vi "Sequencer Main - Copy.vi"() -> ()   [LabVIEW 2018] (continued)
                                frame #0 {
                                n2354 = global read "Global Variable.vi" "COM Port FTDI RS232"() -> (w4643:refnum<visa-resource-name>)
                                n2355 = global read "Global Variable.vi" "Wr PID"() -> (w4640:string)
                                n2356 = call "ADB-Serial_WrRd.vi"("Timeout(Sec)"=1.0, "PassString"=w4640, "Command"="getPID", "ComPort"=w4643) -> ("error out"=w4645:errorcluster, "PASS"=w4646:bool, "received"=w4644:string)  [unwired: 5 in]
                                n2357 = invoke on="Serial CMD Mon" class="Str" method="Append String"("string"=w4644) -> ()  [unwired: 3 in, 4 out]
                                n2358 = Wait (ms)(milliseconds to wait=u32 250) -> ()  [unwired: 1 out]
                                }
                                frame #1 {
                                n2359 = in-place {
                                in-place-border: w4653 -> [w4661]
                                in-place-border: [w4661] -> w4652
                                in-place-border: [w4662] -> w4648
                                in-place-border: w4651 -> [w4659]
                                n2360 = Match Pattern(string=w4659, regular expression="PID:" ("search string/char (-)")) -> (after substring=w4658:string)  [unwired: 1 in, 3 out]
                                n2361 = String Subset(string=w4658, offset (0)=1, length (rest)=13 ("length (rest)")) -> (substring=w4662:string)
                                n2362 = global write "Global Variable.vi" "Rd PID"(w4662) -> ()
                                }
                                n2363 = global read "Global Variable.vi" "Array Errors"() -> (w4657:errorcluster[])
                                n2364 = case shown="False" w4650 {
                                tunnel: [enum16{"Idle", "PASS", "FALSE"}."FALSE" ("Step Test Result") enum16{"Idle", "PASS", "FALSE"}."PASS" ("Step Test Result")] -> w4654
                                frame False {
                                # "Step TEST Result"
                                }
                                frame True {
                                # "Step TEST Result"
                                }
                                }
                                n2365 = Replace Array Subset(array=w4657, new element=w4652, index=3) -> (w4656:errorcluster[])
                                n2366 = global write "Global Variable.vi" "Array Errors"(w4656) -> ()
                                n2367 = Concatenate Strings("Read PID: " ("string"), w4648) -> (w4647:string)
                                }
                              }
                            }
                            frame "setpid" {
                              n2368 = flat-sequence {
                                tunnel: [w4680] -> w4671
                                tunnel: [w4722] -> w4673
                                tunnel: [w4721] -> w4672
                                tunnel: w4671 -> [w4716]
                                tunnel: [w4718] -> w4669
                                tunnel: [w4717] -> w4667
                                frame #0 {
                                w4691 = 5
                                # "Replace Space to 0"
                                # "YY: Year 00-99\nWW: Week 01-53\nSS: Supplier ID (SVI: 04)\nxx: Spare\nNNNNN: Ser Number"
                                # "default"
                                n2369 = local read "Barcode"() -> (w4679:string)
                                n2370 = global write "Global Variable.vi" "Wr PID"("") -> ()
                                n2371 = String Length(string=w4679) -> (length=w4690:i32)
                                n2372 = Greater?(x=w4690, y=w4691) -> (0:w4692:bool)
                                n2373 = case shown="True" w4692 {
                                tunnel: w4679 -> [_ w4715]
                                tunnel: w4691 -> [_ w4713]
                                tunnel: w4690 -> [_ w4714]
                                tunnel: "1111040011111" ("ADB_PID") -> [w4695 w4711]
                                tunnel: [w4695 w4701] -> w4685
                                frame False {
                                }
                                frame True {
                                w4697 = "%2d" ("format string")
                                n2374 = Subtract(x=w4714, y=w4713) -> (x-y=w4712:i32)
                                n2375 = call "Calc_ISO_WeekNumber.vi"() -> ("ISO week number"=w4696:i32, "SBZ year 2 digits"=w4700:i32)  [unwired: 5 in, 5 out]
                                n2376 = String Subset(string=w4715, offset (0)=w4712, length (rest)=w4713) -> (substring=w4710:string)
                                n2377 = Format Into String(format string=w4697, w4700) -> (resulting string=w4699:string)  [unwired: 2 in, 1 out]
                                n2378 = Replace Substring(2:5 ("length (len. of substring)"), 3:8 ("offset (0)"), 4:w4710, 5:w4711) -> (1:w4707:string)  [unwired: 1 out]
                                n2379 = Format Into String(format string=w4697, w4696) -> (resulting string=w4698:string)  [unwired: 2 in, 1 out]
                                n2380 = Replace Substring(2:2 ("offset (0)"), 3:0 ("offset (0)"), 4:w4699, 5:w4707) -> (1:w4702:string)  [unwired: 1 out]
                                n2381 = Replace Substring(2:2 ("offset (0)"), 3:2 ("offset (0)"), 4:w4698, 5:w4702) -> (1:w4701:string)  [unwired: 1 out]
                                }
                                }
                                n2382 = local read "Barcode\nDefault"() -> (w4678:bool)
                                n2383 = call <vilib>:"Space Constant.vi"() -> ("String"=w4683:string)
                                n2384 = call <vilib>:"Search and Replace Pattern.vi"("string"=w4685, "regular expression (\"\")"=w4683, "replace string (\"\")"="0" ("replace string (\"\")")) -> ("result string"=w4681:string)  [unwired: 2 in, 1 out]
                                n2385 = case shown="False" w4678 {
                                tunnel: w4681 -> [_ w4694]
                                tunnel: [w4693 w4694] -> w4680
                                tunnel: w4679 -> [w4693 _]
                                frame False {
                                }
                                frame True {
                                }
                                }
                                n2386 = Concatenate Strings("Calculated PID: ", w4680, "\r\n") -> (w4682:string)
                                n2387 = invoke on="Serial CMD Mon" class="Str" method="Append String"("string"=w4682) -> ()  [unwired: 3 in, 4 out]
                                }
                                frame #1 {
                                n2388 = global read "Global Variable.vi" "COM Port FTDI RS232"() -> (w4720:refnum<visa-resource-name>)
                                n2389 = call "ADB-SetPID.vi"("ADB_PID"=w4716, "ComPort"=w4720) -> ("error out"=w4721:errorcluster, "Wr PID"=w4718:string, "PASS"=w4722:bool, "received"=w4717:string)  [unwired: 6 in]
                                n2390 = invoke on="Serial CMD Mon" class="Str" method="Append String"("string"=w4717) -> ()  [unwired: 3 in, 4 out]
                                n2391 = global write "Global Variable.vi" "Wr PID"(w4718) -> ()
                                n2392 = Wait (ms)(milliseconds to wait=u32 5000) -> ()  [unwired: 1 out]
                                }
                              }
                              n2393 = global read "Global Variable.vi" "Array Errors"() -> (w4676:errorcluster[])
                              n2394 = case shown="False" w4673 {
                                tunnel: [enum16{"Idle", "PASS", "FALSE"}."FALSE" ("Step Test Result") enum16{"Idle", "PASS", "FALSE"}."PASS" ("Step Test Result")] -> w4677
                                frame False {
                                # "Step TEST Result"
                                }
                                frame True {
                                # "Step TEST Result"
                                }
                              }
                              n2395 = Replace Array Subset(array=w4676, new element=w4672, index=5) -> (w4675:errorcluster[])
                              n2396 = Concatenate Strings("Write PID: " ("string"), w4669) -> (w4668:string)
                              n2397 = global write "Global Variable.vi" "Array Errors"(w4675) -> ()
                            }
                            frame "recvtest" {
                              # "Param 1-4"
                              # "Cmd"
                              n2398 = flat-sequence {
                                tunnel: [w4758] -> w4742
                                tunnel: [w4757] -> w4741
                                tunnel: [w4756] -> w4740
                                tunnel: w4739 -> [w4755]
                                tunnel: w4738 -> [w4754]
                                tunnel: w4737 -> [w4753]
                                tunnel: w4736 -> [w4752]
                                tunnel: [w4751] -> w4735
                                tunnel: [w4750] -> w4734
                                tunnel: [w4749] -> w4733
                                tunnel: [w4748] -> w4732
                                tunnel: [w4747] -> w4731
                                tunnel: [w4746] -> w4730
                                tunnel: [w4745] -> w4729
                                tunnel: [w4744] -> w4728
                                tunnel: w4742 -> [w4797]
                                tunnel: w4741 -> [w4816]
                                tunnel: [w4817] -> w4727
                                tunnel: w4740 -> [w4795]
                                tunnel: w4735 -> [w4807]
                                tunnel: w4734 -> [w4806]
                                tunnel: w4733 -> [w4805]
                                tunnel: w4732 -> [w4804]
                                tunnel: w4731 -> [w4803]
                                tunnel: w4730 -> [w4802]
                                tunnel: w4729 -> [w4801]
                                tunnel: w4728 -> [w4800]
                                tunnel: [w4796] -> w4726
                                tunnel: [w4795] -> w4725
                                frame #0 {
                                w4743 = "%f" ("format string")
                                n2399 = for {
                                N: 1 -> [_]
                                tunnel: [w4791] -> w4758
                                tunnel: [w4790] -> w4757
                                tunnel: [w4789] -> w4756
                                stop <- w4791 stop-if-true
                                n2400 = global read "Global Variable.vi" "COM Port FTDI RS232"() -> (w4794:refnum<visa-resource-name>)
                                n2401 = call "ADB-Serial_WrRd.vi"("Timeout(Sec)"=5.0, "PassString"="Chuck(3):", "Command"="recvtest", "ComPort"=w4794) -> ("error out"=w4790:errorcluster, "PASS"=w4791:bool, "received"=w4789:string)  [unwired: 5 in]
                                n2402 = invoke on="Serial CMD Mon" class="Str" method="Append String"("string"=w4789) -> ()  [unwired: 3 in, 4 out]
                                }
                                n2403 = in-place {
                                in-place-border: w4755 -> [w4787]
                                in-place-border: [w4783] -> w4751
                                in-place-border: [w4782] -> w4750
                                in-place-border: w4743 -> [w4781]
                                # "max"
                                # "min"
                                # "LMS RX -> k_est"
                                n2404 = Match Pattern(string=w4787, regular expression=":") -> (before substring=w4785:string, after substring=w4784:string)  [unwired: 1 in, 2 out]
                                n2405 = Scan From String(format string=w4781, input string=w4785) -> (output 1=w4783:dbl)  [unwired: 3 in, 3 out]
                                n2406 = Scan From String(format string=w4781, input string=w4784) -> (output 1=w4782:dbl)  [unwired: 3 in, 3 out]
                                }
                                n2407 = in-place {
                                in-place-border: w4754 -> [w4780]
                                in-place-border: [w4776] -> w4749
                                in-place-border: [w4775] -> w4748
                                in-place-border: w4743 -> [w4774]
                                # "max"
                                # "min"
                                # "LMS RX -> I_est"
                                n2408 = Match Pattern(string=w4780, regular expression=":") -> (before substring=w4778:string, after substring=w4777:string)  [unwired: 1 in, 2 out]
                                n2409 = Scan From String(format string=w4774, input string=w4778) -> (output 1=w4776:dbl)  [unwired: 3 in, 3 out]
                                n2410 = Scan From String(format string=w4774, input string=w4777) -> (output 1=w4775:dbl)  [unwired: 3 in, 3 out]
                                }
                                n2411 = in-place {
                                in-place-border: w4753 -> [w4773]
                                in-place-border: [w4769] -> w4747
                                in-place-border: [w4768] -> w4746
                                in-place-border: w4743 -> [w4767]
                                # "max"
                                # "min"
                                # "CURRENT -> k_est"
                                n2412 = Match Pattern(string=w4773, regular expression=":") -> (before substring=w4771:string, after substring=w4770:string)  [unwired: 1 in, 2 out]
                                n2413 = Scan From String(format string=w4767, input string=w4771) -> (output 1=w4769:dbl)  [unwired: 3 in, 3 out]
                                n2414 = Scan From String(format string=w4767, input string=w4770) -> (output 1=w4768:dbl)  [unwired: 3 in, 3 out]
                                }
                                n2415 = in-place {
                                in-place-border: w4752 -> [w4766]
                                in-place-border: [w4763] -> w4745
                                in-place-border: [w4762] -> w4744
                                in-place-border: w4743 -> [w4761]
                                # "max"
                                # "min"
                                # "CURRENT -> I_est"
                                n2416 = Match Pattern(string=w4766, regular expression=":") -> (before substring=w4765:string, after substring=w4764:string)  [unwired: 1 in, 2 out]
                                n2417 = Scan From String(format string=w4761, input string=w4765) -> (output 1=w4763:dbl)  [unwired: 3 in, 3 out]
                                n2418 = Scan From String(format string=w4761, input string=w4764) -> (output 1=w4762:dbl)  [unwired: 3 in, 3 out]
                                }
                                }
                                frame #1 {
                                n2419 = Match Pattern(string=w4795, regular expression="CURRENT:") -> (after substring=w4798:string, offset past match=w4812:i32)  [unwired: 1 in, 2 out]
                                n2420 = Match Pattern(string=w4795, regular expression="LMS_RX:") -> (after substring=w4799:string, offset past match=w4813:i32)  [unwired: 1 in, 2 out]
                                n2421 = Greater Than 0?(x=w4813) -> (x > 0?=w4810:bool)
                                n2422 = Greater Than 0?(x=w4812) -> (x > 0?=w4811:bool)
                                n2423 = Compound Arithmetic op=AND(w4810, w4811, w4797) -> (w4809:bool)
                                n2424 = case shown="True" w4809 {
                                tunnel: [FALSE w4852] -> w4808
                                tunnel: w4807 -> [_ w4862]
                                tunnel: w4806 -> [_ w4861]
                                tunnel: w4805 -> [_ w4859]
                                tunnel: w4804 -> [_ w4860]
                                tunnel: w4803 -> [_ w4857]
                                tunnel: w4802 -> [_ w4856]
                                tunnel: w4801 -> [_ w4855]
                                tunnel: w4800 -> [_ w4854]
                                tunnel: w4798 -> [_ w4847]
                                tunnel: w4799 -> [_ w4846]
                                tunnel: ["" w4840] -> w4796
                                frame False {
                                }
                                frame True {
                                w4824 = ":" ("string")
                                n2425 = Match Pattern(string=w4846, regular expression="k_est") -> (after substring=w4845:string)  [unwired: 1 in, 3 out]
                                n2426 = Match Pattern(string=w4846, regular expression="l_est") -> (after substring=w4858:string)  [unwired: 1 in, 3 out]
                                n2427 = Match Pattern(string=w4847, regular expression="k_est") -> (after substring=w4833:string)  [unwired: 1 in, 3 out]
                                n2428 = Match Pattern(string=w4847, regular expression="l_est") -> (after substring=w4853:string)  [unwired: 1 in, 3 out]
                                n2429 = call <userlib>:"Multi-line String to Array__ogtk.vi"("string"=w4845) -> ("lines"=w4844:string[])
                                n2430 = call "Loop Test.vi"("Min"=w4862, "Max"=w4861, "Data Str"=w4845) -> ("Result"=w4851:bool)  [unwired: 8 in]
                                n2431 = call "Loop Test.vi"("Min"=w4859, "Max"=w4860, "Data Str"=w4858) -> ("Result"=w4850:bool)  [unwired: 8 in]
                                n2432 = call "Loop Test.vi"("Min"=w4857, "Max"=w4856, "Data Str"=w4833) -> ("Result"=w4849:bool)  [unwired: 8 in]
                                n2433 = call "Loop Test.vi"("Min"=w4855, "Max"=w4854, "Data Str"=w4853) -> ("Result"=w4848:bool)  [unwired: 8 in]
                                n2434 = call <userlib>:"Multi-line String to Array__ogtk.vi"("string"=w4833) -> ("lines"=w4830:string[])
                                n2435 = Index Array(array=w4844, index #1=0, index #2=1) -> (element #1=w4838:string, element #2=w4835:string)
                                n2436 = Index Array(array=w4830, index #1=0, index #2=1) -> (element #1=w4829:string, element #2=w4828:string)
                                n2437 = Compound Arithmetic op=AND(w4851, w4850, w4849, w4848) -> (w4852:bool)
                                n2438 = String Subset(string=w4838, offset (0)=2) -> (substring=w4839:string)  [unwired: 1 in]
                                n2439 = String Subset(string=w4835, offset (0)=7) -> (substring=w4836:string)  [unwired: 1 in]
                                n2440 = String Subset(string=w4829, offset (0)=2) -> (substring=w4825:string)  [unwired: 1 in]
                                n2441 = String Subset(string=w4828, offset (0)=7) -> (substring=w4823:string)  [unwired: 1 in]
                                n2442 = Concatenate Strings(w4839, w4824, w4836, "\r\n", w4825, w4824, w4823) -> (w4840:string)
                                }
                                }
                                n2443 = global read "Global Variable.vi" "Array Errors"() -> (w4820:errorcluster[])
                                n2444 = Replace Array Subset(array=w4820, new element=w4816, index=3) -> (w4819:errorcluster[])
                                n2445 = case shown="False" w4808 {
                                tunnel: [enum16{"Idle", "PASS", "FALSE"}."FALSE" ("Step Test Result") enum16{"Idle", "PASS", "FALSE"}."PASS" ("Step Test Result")] -> w4817
                                frame False {
                                # "Step TEST Result"
                                }
                                frame True {
                                # "Step TEST Result"
                                }
                                }
                                n2446 = global write "Global Variable.vi" "Array Errors"(w4819) -> ()
                                }
                              }
                            }
                            frame "recvtest_2" {
                              # "Param 1-4"
                              # "Cmd"
                              n2447 = flat-sequence {
                                tunnel: [w4885] -> w4878
                                tunnel: [w4884] -> w4877
                                tunnel: [w4883] -> w4876
                                tunnel: w4875 -> [_]
                                tunnel: w4874 -> [_]
                                tunnel: w4873 -> [_]
                                tunnel: w4872 -> [_]
                                tunnel: w4878 -> [w4889]
                                tunnel: w4877 -> [w4890]
                                tunnel: [w4891] -> w4871
                                tunnel: w4876 -> [w4886]
                                tunnel: [w4887] -> w4870
                                tunnel: [w4886] -> w4869
                                frame #0 {
                                n2448 = global read "Global Variable.vi" "COM Port FTDI RS232"() -> (w4882:refnum<visa-resource-name>)
                                n2449 = call "ADB-Serial_WrRd.vi"("Timeout(Sec)"=5.0, "PassString"="Chuck(3):", "Command"="recvtest", "ComPort"=w4882) -> ("error out"=w4884:errorcluster, "PASS"=w4885:bool, "received"=w4883:string)  [unwired: 5 in]
                                n2450 = invoke on="Serial CMD Mon" class="Str" method="Append String"("string"=w4883) -> ()  [unwired: 3 in, 4 out]
                                }
                                frame #1 {
                                n2451 = case shown="True" w4889 {
                                tunnel: w4886 -> [_ w4901]
                                tunnel: [FALSE w4900] -> w4888
                                tunnel: ["Err" ("received") w4899] -> w4887
                                frame False {
                                }
                                frame True {
                                n2452 = Match Pattern(string=w4901, regular expression="TEST SUCCEED") -> (match substring=w4899:string, offset past match=w4898:i32)  [unwired: 1 in, 2 out]
                                n2453 = Greater Than 0?(x=w4898) -> (x > 0?=w4900:bool)
                                }
                                }
                                n2454 = global read "Global Variable.vi" "Array Errors"() -> (w4894:errorcluster[])
                                n2455 = case shown="True" w4888 {
                                tunnel: [enum16{"Idle", "PASS", "FALSE"}."FALSE" ("Step Test Result") enum16{"Idle", "PASS", "FALSE"}."PASS" ("Step Test Result")] -> w4891
                                frame False {
                                # "Step TEST Result"
                                }
                                frame True {
                                # "Step TEST Result"
                                }
                                }
                                n2456 = Replace Array Subset(array=w4894, new element=w4890, index=3) -> (w4893:errorcluster[])
                                n2457 = global write "Global Variable.vi" "Array Errors"(w4893) -> ()
                                }
                              }
                            }
                            frame "readcputemp" {
                              # "Param"
                              # "Cmd"
                              n2458 = flat-sequence {
                                tunnel: [w4918] -> w4910
                                tunnel: [w4916] -> w4908
                                tunnel: [w4917] -> w4906
                                tunnel: [w4916] -> w4904
                                tunnel: w4910 -> [w4928]
                                tunnel: [w4930] -> w4909
                                tunnel: w4908 -> [w4927]
                                tunnel: w4907 -> [w4926]
                                tunnel: w4906 -> [w4925]
                                tunnel: [w4920] -> w4905
                                frame #0 {
                                n2459 = global read "Global Variable.vi" "COM Port FTDI RS232"() -> (w4915:refnum<visa-resource-name>)
                                n2460 = call "ADB-Serial_WrRd.vi"("Timeout(Sec)"=2.0, "PassString"="Chuck(3)", "Command"="readcputemp", "ComPort"=w4915) -> ("error out"=w4917:errorcluster, "PASS"=w4918:bool, "received"=w4916:string)  [unwired: 5 in]
                                n2461 = invoke on="Serial CMD Mon" class="Str" method="Append String"("string"=w4916) -> ()  [unwired: 3 in, 4 out]
                                n2462 = Wait (ms)(milliseconds to wait=u32 300) -> ()  [unwired: 1 out]
                                }
                                frame #1 {
                                n2463 = case shown="True" w4928 {
                                tunnel: [FALSE w4945] -> w4929
                                tunnel: w4927 -> [_ w4942]
                                tunnel: w4926 -> [_ w4941]
                                tunnel: w4925 -> [w4935 w4939]
                                tunnel: [w4935 w4940] -> w4922
                                tunnel: [0.0 w4937] -> w4924
                                frame False {
                                }
                                frame True {
                                n2464 = Match Pattern(string=w4942, regular expression=w4941) -> (after substring=w4938:string)  [unwired: 1 in, 3 out]
                                n2465 = Scan From String(format string="%.; %.3f", input string=w4938, error in=w4939) -> (error out=w4940:errorcluster, output 1=w4937:dbl)  [unwired: 2 in, 2 out]
                                n2466 = Greater Than 0?(x=w4937) -> (x > 0?=w4943:bool)
                                n2467 = case shown="True" w4943 {
                                tunnel: [FALSE TRUE] -> w4945
                                frame False {
                                }
                                frame True {
                                }
                                }
                                }
                                }
                                n2468 = global read "Global Variable.vi" "Array Errors"() -> (w4933:errorcluster[])
                                n2469 = case shown="False" w4929 {
                                tunnel: [enum16{"Idle", "PASS", "FALSE"}."FALSE" ("Step Test Result") enum16{"Idle", "PASS", "FALSE"}."PASS" ("Step Test Result")] -> w4930
                                frame False {
                                # "Step TEST Result"
                                }
                                frame True {
                                # "Step TEST Result"
                                }
                                }
                                n2470 = Format Into String(format string="%.1f C°", initial string="CPU Temp: ", error in=w4922, w4924) -> (resulting string=w4920:string, error out=w4921:errorcluster)
                                n2471 = Replace Array Subset(array=w4933, new element=w4921, index=3) -> (w4932:errorcluster[])
                                n2472 = global write "Global Variable.vi" "Array Errors"(w4932) -> ()
                                }
                              }
                            }
                            frame "up" {
                              # "Param"
                              # "Cmd"
                              n2473 = flat-sequence {
                                tunnel: [w4962] -> w4955
                                tunnel: [w4961] -> w4954
                                tunnel: [w4960] -> w4952
                                tunnel: w4955 -> [w4965]
                                tunnel: w4954 -> [w4967]
                                tunnel: [w4968] -> w4953
                                tunnel: w4952 -> [w4963]
                                tunnel: [w4964] -> w4951
                                tunnel: [w4963] -> w4950
                                frame #0 {
                                n2474 = global read "Global Variable.vi" "COM Port FTDI RS232"() -> (w4959:refnum<visa-resource-name>)
                                n2475 = call "ADB-Serial_WrRd.vi"("Timeout(Sec)"=1.0, "PassString"="Totally", "Command"="up", "ComPort"=w4959) -> ("error out"=w4961:errorcluster, "PASS"=w4962:bool, "received"=w4960:string)  [unwired: 5 in]
                                n2476 = invoke on="Serial CMD Mon" class="Str" method="Append String"("string"=w4960) -> ()  [unwired: 3 in, 4 out]
                                }
                                frame #1 {
                                n2477 = case shown="True" w4965 {
                                tunnel: [FALSE w4981] -> w4966
                                tunnel: w4963 -> [_ w4975]
                                tunnel: ["" w4974] -> w4964
                                frame False {
                                }
                                frame True {
                                n2478 = Match Pattern(string=w4975, regular expression="Totally") -> (after substring=w4978:string)  [unwired: 1 in, 3 out]
                                n2479 = Scan From String(format string="%d", input string=w4978) -> (output 1=w4976:i32)  [unwired: 3 in, 3 out]
                                n2480 = Not Equal To 0?(x=w4976) -> (x != 0?=w4980:bool)
                                n2481 = case shown="True" w4980 {
                                tunnel: [FALSE TRUE] -> w4981
                                tunnel: w4975 -> [_ w4986]
                                tunnel: ["" w4984] -> w4974
                                frame False {
                                }
                                frame True {
                                n2482 = xnode "Match Regular Expression"("input string"=w4986, "regular expression"="\\((.*)\\)") -> ("submatch 1"=w4984:string)  [unwired: 4 in, 5 out]
                                }
                                }
                                }
                                }
                                n2483 = global read "Global Variable.vi" "Array Errors"() -> (w4971:errorcluster[])
                                n2484 = case shown="True" w4966 {
                                tunnel: [enum16{"Idle", "PASS", "FALSE"}."FALSE" ("Step Test Result") enum16{"Idle", "PASS", "FALSE"}."PASS" ("Step Test Result")] -> w4968
                                frame False {
                                # "Step TEST Result"
                                }
                                frame True {
                                # "Step TEST Result"
                                }
                                }
                                n2485 = Replace Array Subset(array=w4971, new element=w4967, index=3) -> (w4970:errorcluster[])
                                n2486 = global write "Global Variable.vi" "Array Errors"(w4970) -> ()
                                }
                              }
                            }
                            frame "readvolt" {
                              # "Param"
                              # "Cmd"
                              n2487 = flat-sequence {
                                tunnel: [w5153] -> w5131
                                tunnel: [w5152] -> w5130
                                tunnel: [w5151] -> w5128
                                tunnel: [w5151] -> w5106
                                tunnel: w5131 -> [w5171]
                                tunnel: w5130 -> [w5172]
                                tunnel: w5128 -> [w5154]
                                tunnel: w5127 -> [w5162]
                                tunnel: w5120 -> [w5170]
                                tunnel: w5121 -> [w5169]
                                tunnel: w5110 -> [w5156]
                                tunnel: w5109 -> [w5159]
                                tunnel: [w5155] -> w5113
                                tunnel: [w5173] -> w5108
                                tunnel: [w5155] -> w5107
                                tunnel: [w5195] -> w5114
                                tunnel: [w5196] -> w5129
                                tunnel: w5108 -> [w5196]
                                tunnel: w5107 -> [w5195]
                                frame #0 {
                                n2488 = global read "Global Variable.vi" "COM Port FTDI RS232"() -> (w5150:refnum<visa-resource-name>)
                                n2489 = call "ADB-Serial_WrRd.vi"("Timeout(Sec)"=1.0, "PassString"="Voltages", "Command"="readvolt", "ComPort"=w5150) -> ("error out"=w5152:errorcluster, "PASS"=w5153:bool, "received"=w5151:string)  [unwired: 5 in]
                                n2490 = invoke on="Serial CMD Mon" class="Str" method="Append String"("string"=w5151) -> ()  [unwired: 3 in, 4 out]
                                }
                                frame #1 {
                                w5164 = "\r\n"
                                w5157 = ">"
                                w5158 = "<"
                                w5166 = "\r\n"
                                w5165 = "******************************************" ("string")
                                n2491 = global read "Global Variable.vi" "Array Errors"() -> (w5176:errorcluster[])
                                n2492 = case shown="True" w5171 {
                                tunnel: w5154 -> [_ w5187]
                                tunnel: w5162 -> [_ w5183]
                                tunnel: w5170 -> [_ w5182]
                                tunnel: w5169 -> [_ w5181]
                                tunnel: [FALSE w5180] -> w5168
                                tunnel: [0 ("Numeric") w5179] -> w5167
                                frame False {
                                }
                                frame True {
                                n2493 = Match Pattern(string=w5187, regular expression=w5183) -> (after substring=w5185:string, offset past match=w5186:i32)  [unwired: 1 in, 2 out]
                                n2494 = Greater Than 0?(x=w5186) -> (x > 0?=w5184:bool)
                                n2495 = case shown="False" w5184 {
                                tunnel: w5185 -> [_ w5192]
                                tunnel: [-9999 ("Numeric") w5189] -> w5179
                                frame False {
                                }
                                frame True {
                                n2496 = Scan From String(format string="%d", input string=w5192, initial scan location=u32 1) -> (output 1=w5189:i32)  [unwired: 2 in, 3 out]
                                }
                                }
                                n2497 = In Range and Coerce(upper limit=w5182, x=w5179, lower limit=w5181) -> (In Range?=w5180:bool)  [unwired: 1 out]
                                }
                                }
                                n2498 = Replace Array Subset(array=w5176, new element=w5172, index=3) -> (w5175:errorcluster[])
                                n2499 = global write "Global Variable.vi" "Array Errors"(w5175) -> ()
                                n2500 = Number To Decimal String(number=w5167) -> (decimal integer string=w5155:string)  [unwired: 1 in]
                                n2501 = Concatenate Strings(w5162, "::") -> (w5163:string)
                                n2502 = Concatenate Strings(w5166, w5165, w5166, w5163, w5158, w5159, w5157, w5158, w5155, w5157, w5158, w5156, w5157, w5164, w5165, w5164) -> (w5160:string)
                                n2503 = case shown="False" w5168 {
                                tunnel: [enum16{"Idle", "PASS", "FALSE"}."FALSE" ("Step Test Result") enum16{"Idle", "PASS", "FALSE"}."PASS" ("Step Test Result")] -> w5173
                                frame False {
                                # "Step TEST Result"
                                }
                                frame True {
                                # "Step TEST Result"
                                }
                                }
                                n2504 = invoke on="Serial CMD Mon" class="Str" method="Append String"("string"=w5160) -> ()  [unwired: 3 in, 4 out]
                                }
                                frame #2 {
                                }
                              }
                              n2505 = global read "Global Variable.vi" "Array_Measurement"() -> (w5125:dbl[])
                              n2506 = Decimal String To Number(string=w5115) -> (number=w5126:i32)  [unwired: 2 in, 1 out]
                              n2507 = Index Array(array=w5125, index=w5126) -> (element=w5124:dbl)
                              n2508 = in-place {
                                in-place-border: w5124 -> [w5144]
                                in-place-border: [w5142] -> w5123
                                in-place-border: [w5139] -> w5122
                                w5140 = 1000.0 ("y")
                                # "Calculate +-3%"
                                n2509 = Multiply(x=w5144, y=1.03) -> (x*y=w5145:dbl)
                                n2510 = Multiply(x=w5144, y=0.97) -> (x*y=w5141:dbl)
                                n2511 = Multiply(x=w5145, y=w5140) -> (x*y=w5142:dbl)
                                n2512 = Multiply(x=w5140, y=w5141) -> (x*y=w5139:dbl)
                              }
                              n2513 = To Unsigned Long Integer(number=w5123) -> (unsigned 32bit integer=w5120:u32)
                              n2514 = To Unsigned Long Integer(number=w5122) -> (unsigned 32bit integer=w5121:u32)
                              n2515 = Number To Decimal String(number=w5120) -> (decimal integer string=w5118:string)  [unwired: 1 in]
                              n2516 = Number To Decimal String(number=w5121) -> (decimal integer string=w5116:string)  [unwired: 1 in]
                              n2517 = Concatenate Strings("max " ("string"), w5118) -> (w5110:string)
                              n2518 = Concatenate Strings("min " ("string"), w5116) -> (w5109:string)
                              n2519 = Concatenate Strings(w5110, "\r\n", w5109) -> (w5111:string)
                              n2520 = in-place {
                                in-place-border: w5113 -> [w5134]
                                in-place-border: w5111 -> [w5132]
                                # "Set Parameters to \nTest Seguenser Table"
                                n2521 = global read "Global Variable.vi" "Current Step Nmb"() -> (w5136:u32)
                                n2522 = property on="Test Squencer Edit" class="MCListbox (strict)"() -> ("ItemNames"=w5138:string[][])  [unwired: 2 in, 2 out]
                                n2523 = Replace Array Subset(array=w5138, new element #1=w5134, index (row) #1=w5136, index (col) #1=2 ("disabled index (col)"), new element #2=w5132, index (row) #2=w5136, index (col) #2=4 ("disabled index (col)")) -> (w5137:string[][])
                                n2524 = property on="Test Squencer Edit" class="MCListbox (strict)"("ItemNames"=w5137) -> ()  [unwired: 2 in, 2 out]
                              }
                            }
                            frame "capmem" {
                              w5203 = "max: "
                              w5204 = ">" ("string")
                              w5206 = "<" ("string")
                              w5208 = "min: "
                              # "Parameters"
                              # "Cmd"
                              n2525 = flat-sequence {
                                tunnel: [w5240] -> w5226
                                tunnel: [w5239] -> w5225
                                tunnel: [w5238] -> w5197
                                tunnel: w5226 -> [w5273]
                                tunnel: w5225 -> [w5274]
                                tunnel: w5222 -> [w5272]
                                tunnel: w5217 -> [w5271]
                                tunnel: w5221 -> [w5269]
                                tunnel: w5220 -> [w5268]
                                tunnel: [w5267] -> w5213
                                tunnel: [w5270] -> w5199
                                tunnel: [w5349] -> w5198
                                tunnel: w5199 -> [w5349]
                                frame #0 {
                                n2526 = for {
                                N: 1 -> [_]
                                tunnel: [w5245] -> w5240
                                tunnel: [w5244] -> w5239
                                tunnel: [w5242] -> w5238
                                i -> [w5243]
                                n2527 = case shown="1" w5243 {
                                tunnel: [w5251 w5263] -> w5245
                                tunnel: [w5247 w5256] -> w5244
                                tunnel: [w5246 w5255] -> w5242
                                frame 0, Default {
                                n2528 = global read "Global Variable.vi" "COM Port FTDI RS232"() -> (w5254:refnum<visa-resource-name>)
                                n2529 = call "ADB-Serial_WrRd.vi"("Timeout(Sec)"=2.0, "PassString"="Chuck(3)", "Command"="capmem 1", "ComPort"=w5254) -> ("error out"=w5248:errorcluster, "PASS"=w5251:bool, "received"=w5246:string)  [unwired: 5 in]
                                n2530 = invoke on="Serial CMD Mon" class="Str" method="Append String"(error in=w5248, "string"=w5246) -> (error out=w5247:errorcluster)  [unwired: 2 in, 3 out]
                                n2531 = Wait (ms)(milliseconds to wait=u32 1000) -> ()  [unwired: 1 out]
                                }
                                frame 1 {
                                w5258 = "\r\n"
                                n2532 = global read "Global Variable.vi" "COM Port FTDI RS232"() -> (w5266:refnum<visa-resource-name>)
                                n2533 = call "ADB-Serial_WrRd.vi"("Timeout(Sec)"=2.0, "PassString"="Chuck(3)", "Command"="capmem 0", "ComPort"=w5266) -> ("error out"=w5257:errorcluster, "PASS"=w5263:bool, "received"=w5255:string)  [unwired: 5 in]
                                n2534 = Concatenate Strings(w5255, w5258, "DELAY->5Sec", w5258) -> (w5260:string)
                                n2535 = invoke on="Serial CMD Mon" class="Str" method="Append String"(error in=w5257, "string"=w5260) -> (error out=w5256:errorcluster)  [unwired: 2 in, 3 out]
                                n2536 = Wait (ms)(milliseconds to wait=u32 4500) -> ()  [unwired: 1 out]
                                }
                                }
                                }
                                }
                                frame #1 {
                                n2537 = case shown="True" w5273 {
                                tunnel: w5272 -> [_ w5291]
                                tunnel: w5271 -> [_ w5290]
                                tunnel: [enum16{"Idle", "PASS", "FALSE"}."FALSE" ("Step Test Result") w5289] -> w5270
                                tunnel: w5269 -> [_ w5288]
                                tunnel: w5268 -> [_ w5287]
                                tunnel: [i32[] [0, 0] w5280] -> w5267
                                frame False {
                                }
                                frame True {
                                n2538 = for {
                                N: 2 -> [_]
                                tunnel: w5291 -> [w5300]
                                tunnel: w5290 -> [w5299]
                                tunnel: w5288 -> [w5298]
                                tunnel: w5287 -> [w5297]
                                tunnel: [w5296] -> w5286 mode=indexing
                                tunnel: [w5295] -> w5280 mode=indexing
                                i -> [w5301]
                                n2539 = case shown="1" w5301 {
                                tunnel: w5300 -> [w5316 _]
                                tunnel: w5299 -> [w5315 _]
                                tunnel: w5298 -> [_ w5333]
                                tunnel: w5297 -> [_ w5332]
                                tunnel: [w5309 w5331] -> w5296
                                tunnel: [w5302 w5327] -> w5295
                                frame 0, Default {
                                w5305 = "\r\n"
                                n2540 = global read "Global Variable.vi" "COM Port FTDI RS232"() -> (w5322:refnum<visa-resource-name>)
                                n2541 = Wait (ms)(milliseconds to wait=u32 4500) -> ()  [unwired: 1 out]
                                n2542 = call "ADB-Serial_WrRd.vi"("Timeout(Sec)"=3.0, "PassString"="Chuck(3)", "Command"="capmem", "ComPort"=w5322) -> ("error out"=w5304:errorcluster, "PASS"=w5310:bool, "received"=w5307:string)  [unwired: 5 in]
                                n2543 = property on="Msg Str" class="Str"("Text.Scroll Position"=inf) -> ()  [unwired: 2 in, 2 out]
                                n2544 = Match Pattern(string=w5307, regular expression="voltage") -> (after substring=w5320:string)  [unwired: 1 in, 3 out]
                                n2545 = Concatenate Strings(w5307, w5305, "DELAY->5Sec", w5305) -> (w5308:string)
                                n2546 = Scan From String(format string="%d", input string=w5320, initial scan location=u32 0) -> (output 1=w5302:i32)  [unwired: 2 in, 3 out]
                                n2547 = global read "Global Variable.vi" "Array Errors"() -> (w5312:errorcluster[])
                                n2548 = In Range and Coerce(upper limit=w5316, x=w5302, lower limit=w5315) -> (In Range?=w5311:bool)  [unwired: 1 out]
                                n2549 = invoke on="Serial CMD Mon" class="Str" method="Append String"(error in=w5304, "string"=w5308) -> (error out=w5303:errorcluster)  [unwired: 2 in, 3 out]
                                n2550 = Replace Array Subset(array=w5312, new element=w5303, index=3) -> (w5313:errorcluster[])
                                n2551 = And(x=w5311, y=w5310) -> (x .and. y?=w5309:bool)
                                n2552 = global write "Global Variable.vi" "Array Errors"(w5313) -> ()
                                }
                                frame 1 {
                                n2553 = global read "Global Variable.vi" "COM Port FTDI RS232"() -> (w5344:refnum<visa-resource-name>)
                                n2554 = call "ADB-Serial_WrRd.vi"("Timeout(Sec)"=3.0, "PassString"="Chuck(3)", "Command"="capmem", "ComPort"=w5344) -> ("error out"=w5329:errorcluster, "PASS"=w5334:bool, "received"=w5330:string)  [unwired: 5 in]
                                n2555 = invoke on="Serial CMD Mon" class="Str" method="Append String"("string"=w5330) -> ()  [unwired: 3 in, 4 out]
                                n2556 = property on="Msg Str" class="Str"(error in=w5329, "Text.Scroll Position"=inf) -> (error out=w5328:errorcluster)  [unwired: 1 in, 1 out]
                                n2557 = Match Pattern(string=w5330, regular expression="voltage") -> (after substring=w5342:string)  [unwired: 1 in, 3 out]
                                n2558 = Scan From String(format string="%d", input string=w5342, initial scan location=u32 0) -> (output 1=w5327:i32)  [unwired: 2 in, 3 out]
                                n2559 = global read "Global Variable.vi" "Array Errors"() -> (w5336:errorcluster[])
                                n2560 = In Range and Coerce(upper limit=w5333, x=w5327, lower limit=w5332) -> (In Range?=w5335:bool)  [unwired: 1 out]
                                n2561 = Replace Array Subset(array=w5336, new element=w5328, index=3) -> (w5337:errorcluster[])
                                n2562 = global write "Global Variable.vi" "Array Errors"(w5337) -> ()
                                n2563 = And(x=w5335, y=w5334) -> (x .and. y?=w5331:bool)
                                n2564 = Wait (ms)(milliseconds to wait=u32 1000) -> ()  [unwired: 1 out]
                                }
                                }
                                }
                                n2565 = Index Array(array=w5286, index #1=0 ("index"), index #2=1 ("index")) -> (element #1=w5285:bool, element #2=w5284:bool)
                                n2566 = And(x=w5285, y=w5284) -> (x .and. y?=w5283:bool)
                                n2567 = case shown="True" w5283 {
                                tunnel: [enum16{"Idle", "PASS", "FALSE"}."FALSE" ("Step Test Result") enum16{"Idle", "PASS", "FALSE"}."PASS" ("Step Test Result")] -> w5289
                                frame False {
                                # "Step TEST Result"
                                }
                                frame True {
                                # "Step TEST Result"
                                }
                                }
                                }
                                }
                                n2568 = global read "Global Variable.vi" "Array Errors"() -> (w5277:errorcluster[])
                                n2569 = Replace Array Subset(array=w5277, new element=w5274, index=3) -> (w5276:errorcluster[])
                                n2570 = global write "Global Variable.vi" "Array Errors"(w5276) -> ()
                                }
                                frame #2 {
                                }
                              }
                              n2571 = in-place {
                                in-place-border: w5224 -> [w5237]
                                in-place-border: w5223 -> [w5236]
                                in-place-border: [w5234] -> w5222
                                in-place-border: [w5233] -> w5217
                                in-place-border: [w5232] -> w5221
                                in-place-border: [w5231] -> w5220
                                in-place-border: [w5228] -> w5216
                                in-place-border: [w5227] -> w5210
                                in-place-border: [w5230] -> w5207
                                in-place-border: [w5229] -> w5202
                                w5235 = "-"
                                # "param-2 : min / max"
                                # "param-1 : min / max"
                                n2572 = Match Pattern(string=w5237, regular expression=w5235) -> (before substring=w5227:string, after substring=w5228:string)  [unwired: 1 in, 2 out]
                                n2573 = Match Pattern(string=w5236, regular expression=w5235) -> (before substring=w5229:string, after substring=w5230:string)  [unwired: 1 in, 2 out]
                                n2574 = Decimal String To Number(string=w5228) -> (number=w5233:i32)  [unwired: 2 in, 1 out]
                                n2575 = Decimal String To Number(string=w5230) -> (number=w5231:i32)  [unwired: 2 in, 1 out]
                                n2576 = Decimal String To Number(string=w5227) -> (number=w5234:i32)  [unwired: 2 in, 1 out]
                                n2577 = Decimal String To Number(string=w5229) -> (number=w5232:i32)  [unwired: 2 in, 1 out]
                              }
                              n2578 = Index Array(array=w5213, index #1=0, index #2=1) -> (element #1=w5201:i32, element #2=w5211:i32)
                              n2579 = Number To Decimal String(number=w5201) -> (decimal integer string=w5212:string)  [unwired: 1 in]
                              n2580 = Number To Decimal String(number=w5211) -> (decimal integer string=w5205:string)  [unwired: 1 in]
                              n2581 = Concatenate Strings("Delay-5S -> ", w5208, w5216, w5206, w5212, w5204, w5203, w5210, "\r\n", "Delay-5S -> ", w5208, w5207, w5206, w5205, w5204, w5203, w5202) -> (w5218:string)
                            }
                            frame "capmem_set" {
                              # "Need 2 Times!"
                              # "Parameters"
                              # "Cmd"
                              n2582 = flat-sequence {
                                tunnel: [w5364] -> w5355
                                tunnel: [w5363] -> w5354
                                tunnel: [w5356] -> w5350
                                tunnel: w5355 -> [w5391]
                                tunnel: w5354 -> [w5392]
                                tunnel: [w5390] -> w5353
                                tunnel: [w5389] -> w5351
                                tunnel: w5350 -> [w5389]
                                frame #0 {
                                w5357 = "\r\n"
                                n2583 = for {
                                N: 2 -> [_]
                                tunnel: [w5369] -> w5364
                                tunnel: [w5368] -> w5363
                                tunnel: [w5366] -> w5362 mode=indexing
                                i -> [w5367]
                                n2584 = case shown="1" w5367 {
                                tunnel: [w5375 w5385] -> w5369
                                tunnel: [w5371 w5380] -> w5368
                                tunnel: [w5370 w5379] -> w5366
                                frame 0, Default {
                                n2585 = global read "Global Variable.vi" "COM Port FTDI RS232"() -> (w5378:refnum<visa-resource-name>)
                                n2586 = call "ADB-Serial_WrRd.vi"("Timeout(Sec)"=1.0, "PassString"="Chuck(3)", "Command"="capmem 1", "ComPort"=w5378) -> ("error out"=w5372:errorcluster, "PASS"=w5375:bool, "received"=w5370:string)  [unwired: 5 in]
                                n2587 = invoke on="Serial CMD Mon" class="Str" method="Append String"(error in=w5372, "string"=w5370) -> (error out=w5371:errorcluster)  [unwired: 2 in, 3 out]
                                n2588 = Wait (ms)(milliseconds to wait=u32 1000) -> ()  [unwired: 1 out]
                                }
                                frame 1 {
                                n2589 = global read "Global Variable.vi" "COM Port FTDI RS232"() -> (w5388:refnum<visa-resource-name>)
                                n2590 = call "ADB-Serial_WrRd.vi"("Timeout(Sec)"=1.0, "PassString"="Chuck(3)", "Command"="capmem 0", "ComPort"=w5388) -> ("error out"=w5381:errorcluster, "PASS"=w5385:bool, "received"=w5379:string)  [unwired: 5 in]
                                n2591 = Concatenate Strings(w5379, "\r\n") -> (w5383:string)
                                n2592 = invoke on="Serial CMD Mon" class="Str" method="Append String"(error in=w5381, "string"=w5383) -> (error out=w5380:errorcluster)  [unwired: 2 in, 3 out]
                                }
                                }
                                }
                                n2593 = Index Array(array=w5362, index #1=0 ("index"), index #2=1 ("index")) -> (element #1=w5359:string, element #2=w5358:string)
                                n2594 = Concatenate Strings(w5359, w5357, w5358, w5357) -> (w5356:string)
                                }
                                frame #1 {
                                n2595 = case shown="True" w5391 {
                                tunnel: [enum16{"Idle", "PASS", "FALSE"}."FALSE" ("Step Test Result") enum16{"Idle", "PASS", "FALSE"}."PASS" ("Step Test Result")] -> w5390
                                frame False {
                                }
                                frame True {
